vi "SR6-NC Inverse Kinematics.vi"(8 "error in (no error)":errorcluster, 10 "end effector transform":T1, 11 "SR6-NC Arm in":refnum<class "SR6-NC Arm.lvclass">) -> (0 "error out":errorcluster, 1 "number of valid solutions":i32, 2 "joint positions":T1, 3 "SR6-NC Arm out":refnum<class "SR6-NC Arm.lvclass">)   [LabVIEW 2013, in "SR6-NC Arm.lvclass"]
uses:
  SR6-NC Arm.lvclass
  <vilib>/Analysis/Matrix/Datatypes/RealMatrix.ctl
  <vilib>/robotics/Kinematics/Link/NI_Robotics_Link.lvclass/NI_Robotics_Link.ctl
  <vilib>/Analysis/baseanly.llb/Real A x B.vi
  <vilib>/Analysis/baseanly.llb/A x Vector.vi
  <vilib>/Analysis/coordinate.llb/Wrap Angle (scalar).vi
  <vilib>/Analysis/_algsub.llb/Real Vector Norm.vi
  <vilib>/Analysis/7linalg.llb/Real Transpose Matrix.vi
  <vilib>/Analysis/baseanly.llb/Real Inverse Matrix.vi
  <vilib>/robotics/Kinematics/Robot/NI_Robotics_Serial Robot Arm.lvclass
  <vilib>/robotics/Kinematics/Link/NI_Robotics_Link.lvclass
  <vilib>/Analysis/NI_AALBase.lvlib
  <vilib>/robotics/Kinematics/NI_Kinematics.lvlib
  <vilib>/Analysis/NI_AALPro.lvlib
  <vilib>/Analysis/NI_AAL_Angle.lvlib
  <vilib>/Analysis/coordinate.llb/Euler Rotation Order.ctl
  <vilib>/Analysis/Matrix/NI_Matrix.lvlib
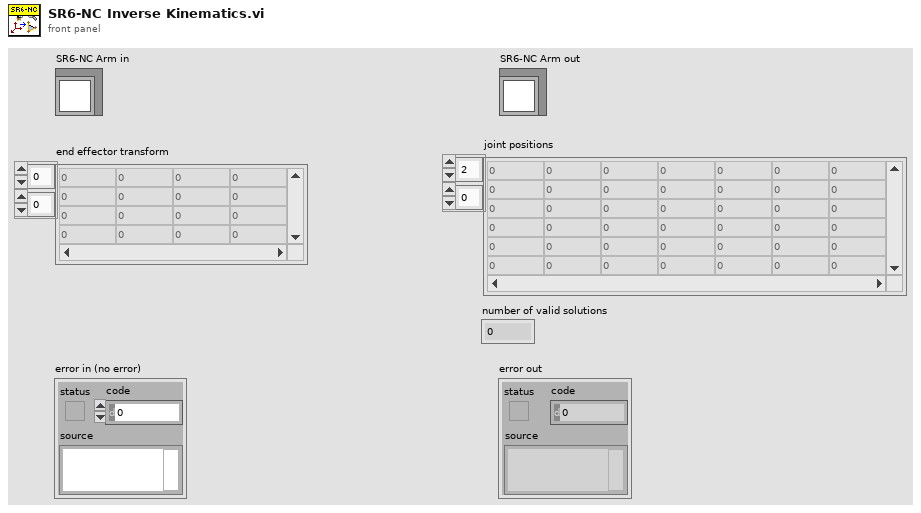
[diagram p1: front panel]
types:
  T1 = typedef "NI_Matrix.lvlib/RealMatrix.ctl" = dbl[][]
  T2 = typedef "NI_AALPro.lvlib/Euler Rotation Order.ctl" = u16
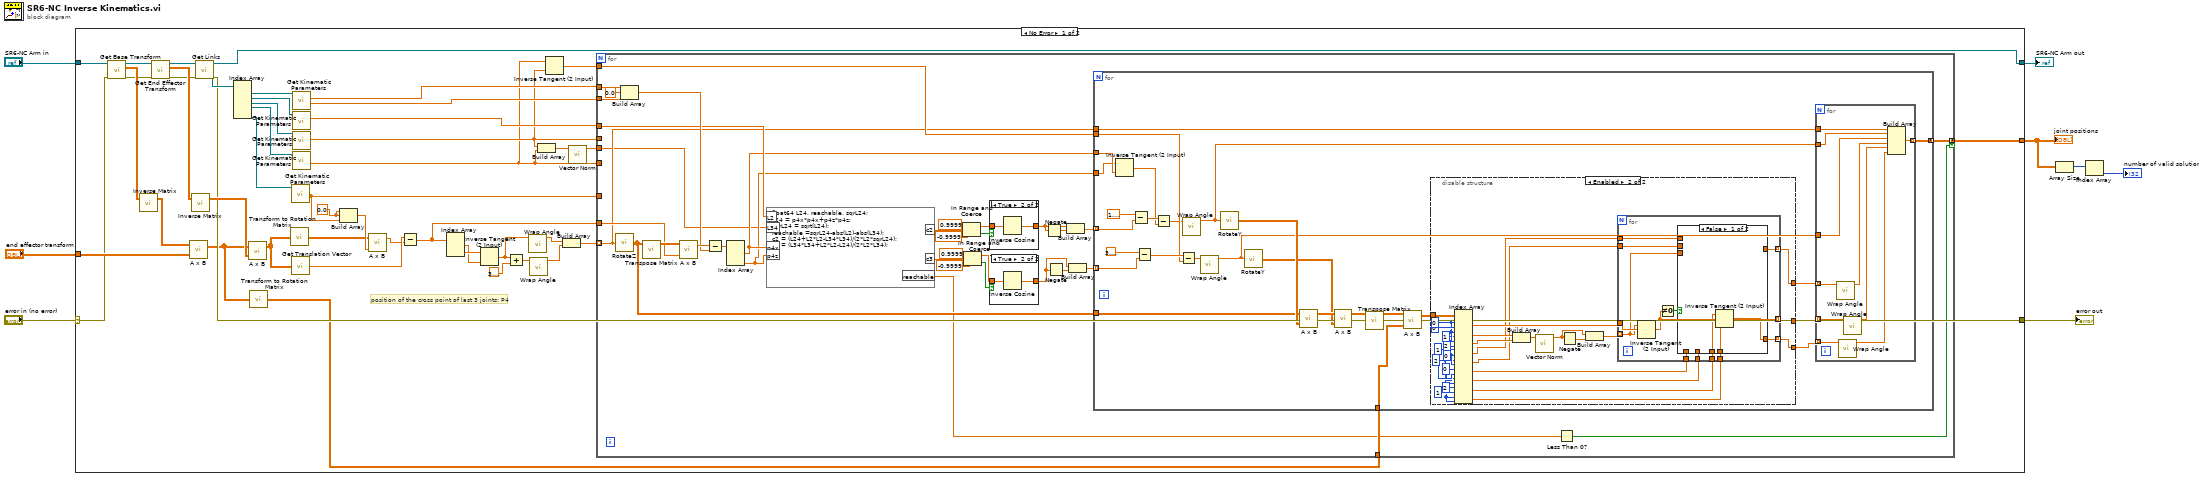
[diagram p0: block diagram]
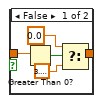
[diagram p2: hidden frame]
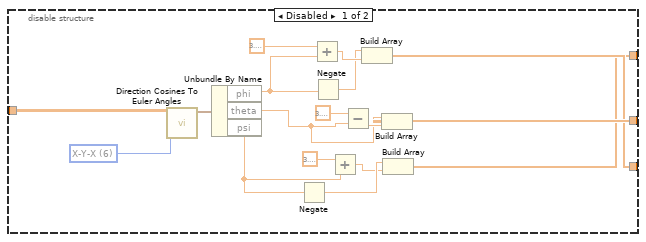
[diagram p3: hidden frame]
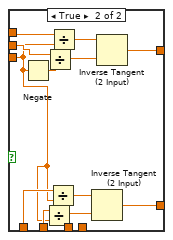
[diagram p4: hidden frame]
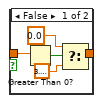
[diagram p5: hidden frame]
diagram:
  n1 = case shown="No Error" "error in (no error)" {
    selector: "error in (no error)" -> [w21 w213]
    tunnel: [w20 w213] -> w7
    tunnel: [w22 w212] -> w5
    tunnel: "SR6-NC Arm in" -> [w52 w212]
    tunnel: "end effector transform" -> [w43 _]
    tunnel: [w23 _] -> w3
    frame No Error {
      w10 = 0.0 ("element")
      # "position of the cross point of last 3 joints: P4"
      n2 = call <vilib>:"Get Base Transform.vi"("error in (no error)"=w21, "serial arm in"=w52) -> ("error out"=w45:errorcluster, "base transform"=w47:T1, "serial arm out"=w51:refnum<class "SR6-NC Arm.lvclass">)  [unwired: 7 in]
      n3 = call-poly <vilib>:"Inverse Matrix.vi"("Input Matrix"=w47) -> ("Inverse Matrix"=w49:T1)  [unwired: 1 in, 1 out]
      n4 = call <vilib>:"Get End Effector Transform.vi"("error in (no error)"=w45, "serial arm in"=w51) -> ("error out"=w44:errorcluster, "end effector transform"=w46:T1, "serial arm out"=w50:refnum<class "SR6-NC Arm.lvclass">)  [unwired: 7 in]
      n5 = call-poly <vilib>:"A x B.vi"("B"=w43, "A"=w49) -> ("A x B"=w12:T1)  [unwired: 1 out]
      n6 = call-poly <vilib>:"Inverse Matrix.vi"("Input Matrix"=w46) -> ("Inverse Matrix"=w48:T1)  [unwired: 1 in, 1 out]
      n7 = call <vilib>:"Get Links.vi"("error in (no error)"=w44, "serial arm in"=w50) -> ("error out"=w20:errorcluster, "links"=w54:refnum<class "NI_Robotics_Link.lvclass">[], "serial arm out"=w22:refnum<class "SR6-NC Arm.lvclass">)  [unwired: 7 in]
      n8 = Index Array(array=w54) -> (element #1=w53:refnum<class "NI_Robotics_Link.lvclass">, element #2=w35:refnum<class "NI_Robotics_Link.lvclass">, element #3=w34:refnum<class "NI_Robotics_Link.lvclass">, element #4=w33:refnum<class "NI_Robotics_Link.lvclass">, element #6=w32:refnum<class "NI_Robotics_Link.lvclass">)  [unwired: 6 in, 1 out]
      n9 = call-poly <vilib>:"A x B.vi"("B"=w48, "A"=w12) -> ("A x B"=w42:T1)  [unwired: 1 out]
      n10 = call <vilib>:"Transform to Rotation Matrix.vi"("transform"=w12) -> ("rotation matrix"=w11:T1)
      n11 = call <vilib>:"Transform to Rotation Matrix.vi"("transform"=w42) -> ("rotation matrix"=w13:T1)
      n12 = call <vilib>:"Get Translation Vector.vi"("transform"=w42) -> ("translation vector"=w30:dbl[])
      n13 = call <vilib>:"Get Kinematic Parameters.vi"("NI_Robotics_Link in"=w32) -> ("Offset Distance"=w9:dbl)  [unwired: 6 in, 4 out]
      n14 = call <vilib>:"Get Kinematic Parameters.vi"("NI_Robotics_Link in"=w35) -> ("Length"=w27:dbl)  [unwired: 6 in, 4 out]
      n15 = call <vilib>:"Get Kinematic Parameters.vi"("NI_Robotics_Link in"=w33) -> ("Offset Distance"=w16:dbl)  [unwired: 6 in, 4 out]
      n16 = call <vilib>:"Get Kinematic Parameters.vi"("NI_Robotics_Link in"=w53) -> ("Offset Distance"=w18:dbl, "Length"=w19:dbl)  [unwired: 6 in, 3 out]
      n17 = call <vilib>:"Get Kinematic Parameters.vi"("NI_Robotics_Link in"=w34) -> ("Length"=w17:dbl)  [unwired: 6 in, 4 out]
      n18 = Build Array(w10, w10, w9) -> (w31:dbl[])
      n19 = call-poly <vilib>:"A x B.vi"("Vector"=w31, "A"=w13) -> ("A x Vector"=w29:dbl[])  [unwired: 1 out]
      n20 = Subtract(x=w30, y=w29) -> (x-y=w28:dbl[])
      n21 = Index Array(array=w28) -> (element #1=w40:dbl, element #2=w41:dbl)  [unwired: 3 in, 1 out]
      n22 = Inverse Tangent (2 Input)(1:w40, 2:w41) -> (0:w24:dbl)
      n23 = Add(x=w24, y=3.141592653589793) -> (x+y=w38:dbl)
      n24 = call-poly <vilib>:"Wrap Angle.vi"("angle in"=w24) -> ("angle out"=w25:dbl)  [unwired: 9 in, 1 out]
      n25 = call-poly <vilib>:"Wrap Angle.vi"("angle in"=w38) -> ("angle out"=w37:dbl)  [unwired: 9 in, 1 out]
      n26 = Build Array(w17, w16) -> (w15:dbl[])
      n27 = Inverse Tangent (2 Input)(1:w17, 2:w16) -> (0:w26:dbl)
      n28 = Build Array(w25, w37) -> (w36:dbl[])
      n29 = call-poly <vilib>:"Vector Norm.vi"("Input Vector"=w15) -> ("norm"=w14:dbl)  [unwired: 9 in, 1 out]
      n30 = for {
        tunnel: w36 -> [w59] mode=indexing
        tunnel: w18 -> [w85]
        tunnel: w19 -> [w86]
        tunnel: w27 -> [w81]
        tunnel: w17 -> [_]
        tunnel: w16 -> [_]
        tunnel: w9 -> [_]
        tunnel: w28 -> [w88]
        tunnel: w26 -> [w62]
        tunnel: w11 -> [w60]
        tunnel: [w58] -> w23 mode=concatenating if=w56
        tunnel: w14 -> [w55]
        n31 = call <vilib>:"RotateZ.vi"("theta"=w59) -> ("rotation matrix"=w61:T1)
        n32 = Build Array(w86, 0.0 ("element"), w85) -> (w83:dbl[])
        n33 = call-poly <vilib>:"Transpose Matrix.vi"("Input Matrix"=w61) -> ("Matrix Transpose"=w89:T1)  [unwired: 9 in, 1 out]
        n34 = call-poly <vilib>:"A x B.vi"("Vector"=w88, "A"=w89) -> ("A x Vector"=w87:dbl[])  [unwired: 1 out]
        n35 = Subtract(x=w87, y=w83) -> (x-y=w82:dbl[])
        n36 = Index Array(array=w82) -> (element #1=w72:dbl, element #3=w71:dbl)  [unwired: 3 in, 1 out]
        n37 = formula code="float64 L24, reachable, sqrL24;\nL24 = p4x*p4x+p4z*p4z;\nsqrL24 = sqrt(L24);\nreachable =sqrL24-abs(L2)-abs(L34);\nc2 = (L24+L2*L2-L34*L34)/(2*L2*sqrL24);\nc3 = (L34*L34+L2*L2-L24)/(2*L2*L34);"("p4x"=w72, "p4z"=w71, "L2"=w81, "L34"=w55) -> ("c2"=w76:dbl, "reachable"=w57:dbl, "c3"=w66:dbl)
        n38 = In Range and Coerce(upper limit=0.9999, x=w76, lower limit=-0.9999) -> (coerced(x)=w77:dbl, In Range?=w78:bool)
        n39 = In Range and Coerce(upper limit=0.9999, x=w66, lower limit=-0.9999) -> (coerced(x)=w67:dbl, In Range?=w68:bool)
        n40 = case shown="True" w78 {
          tunnel: w77 -> [w209 w211]
          tunnel: [w205 w210] -> w74
          frame False {
            n41 = Greater Than 0?(x=w209) -> (x > 0?=w208:bool)
            n42 = Select(t=0.0, s=w208, f=3.141592653589793) -> (s? t:f=w205:dbl)
          }
          frame True {
            n43 = Inverse Cosine(1:w211) -> (0:w210:dbl)
          }
        }
        n44 = case shown="True" w68 {
          tunnel: w67 -> [w94 w96]
          tunnel: [w90 w95] -> w64
          frame False {
            n45 = Greater Than 0?(x=w94) -> (x > 0?=w93:bool)
            n46 = Select(t=0.0, s=w93, f=3.141592653589793) -> (s? t:f=w90:dbl)
          }
          frame True {
            n47 = Inverse Cosine(1:w96) -> (0:w95:dbl)
          }
        }
        n48 = Negate(x=w74) -> (-x=w75:dbl)
        n49 = Negate(x=w64) -> (-x=w65:dbl)
        n50 = Build Array(w74, w75) -> (w73:dbl[])
        n51 = Build Array(w64, w65) -> (w63:dbl[])
        n52 = for {
          tunnel: w73 -> [w122] mode=indexing
          tunnel: w72 -> [w121]
          tunnel: w71 -> [w120]
          tunnel: w63 -> [w116] mode=indexing
          tunnel: w62 -> [w114]
          tunnel: w61 -> [w97]
          tunnel: w60 -> [w108]
          tunnel: w59 -> [w101]
          tunnel: [w98] -> w58 mode=concatenating
          n53 = Inverse Tangent (2 Input)(1:w121, 2:w120) -> (0:w118:dbl)
          n54 = Subtract(x=1.5707963267948966, y=w122) -> (x-y=w119:dbl)
          n55 = Subtract(x=3.141592653589793, y=w116) -> (x-y=w115:dbl)
          n56 = Subtract(x=w119, y=w118) -> (x-y=w106:dbl)
          n57 = Subtract(x=w115, y=w114) -> (x-y=w105:dbl)
          n58 = call-poly <vilib>:"Wrap Angle.vi"("angle in"=w106) -> ("angle out"=w100:dbl)  [unwired: 9 in, 1 out]
          n59 = call-poly <vilib>:"Wrap Angle.vi"("angle in"=w105) -> ("angle out"=w99:dbl)  [unwired: 9 in, 1 out]
          n60 = call <vilib>:"RotateY.vi"("theta"=w100) -> ("rotation matrix"=w113:T1)
          n61 = call <vilib>:"RotateY.vi"("theta"=w99) -> ("rotation matrix"=w111:T1)
          n62 = call-poly <vilib>:"A x B.vi"("B"=w113, "A"=w97) -> ("A x B"=w112:T1)  [unwired: 1 out]
          n63 = call-poly <vilib>:"A x B.vi"("B"=w111, "A"=w112) -> ("A x B"=w110:T1)  [unwired: 1 out]
          n64 = call-poly <vilib>:"Transpose Matrix.vi"("Input Matrix"=w110) -> ("Matrix Transpose"=w109:T1)  [unwired: 9 in, 1 out]
          n65 = call-poly <vilib>:"A x B.vi"("B"=w108, "A"=w109) -> ("A x B"=w107:T1)  [unwired: 1 out]
          n66 = disable-structure shown="Enabled" {
            disable-tunnel: w107 -> [w140 w167]
            disable-tunnel: [w124 w151] -> w104
            disable-tunnel: [w132 w155] -> w103
            disable-tunnel: [w125 w145] -> w102
            frame Disabled {
              w139 = T2 6 items=["X-Y-Z", "X-Z-Y", "Y-X-Z", "Y-Z-X", "Z-X-Y", "Z-Y-X", "X-Y-X", "X-Z-X", "Y-X-Y", "Y-Z-Y", "Z-X-Z", "Z-Y-Z"] ("rotation order")
              n67 = call <vilib>:"Direction Cosines To Euler Angles.vi"("rotation order"=w139, "Direction Cosines"=w140) -> ("Euler Angles"=w138:cluster{"phi":dbl, "theta":dbl, "psi":dbl})  [unwired: 8 in, 1 out]
              n68 = Unbundle By Name(w138) -> ("phi"=w136:dbl, "theta"=w126:dbl, "psi"=w133:dbl)
              n69 = Negate(x=w133) -> (-x=w128:dbl)
              n70 = Add(x=3.141592653589793, y=w136) -> (x+y=w131:dbl)
              n71 = Negate(x=w136) -> (-x=w130:dbl)
              n72 = Add(x=3.141592653589793, y=w133) -> (x+y=w127:dbl)
              n73 = Subtract(x=3.141592653589793, y=w126) -> (x-y=w129:dbl)
              n74 = Build Array(w130, w131) -> (w125:dbl[])
              n75 = Build Array(w126, w129) -> (w132:dbl[])
              n76 = Build Array(w128, w127) -> (w124:dbl[])
            }
            frame Enabled {
              w143 = 2 ("index (row)")
              w149 = 0 ("index (row)")
              w148 = 2 ("index (row)")
              w154 = 0 ("disabled index (col)")
              w150 = 1 ("index (row)")
              w165 = 0 ("index (row)")
              n77 = Index Array(array=w167, index (row) #1=w165, index (col) #1=0 ("disabled index (col)"), index (row) #2=w165, index (col) #2=1 ("disabled index (col)"), index (row) #3=w165, index (col) #3=2 ("disabled index (col)"), index (row) #4=w150, index (col) #4=w154, index (row) #5=w148, index (col) #5=w154, index (row) #6=w149, index (col) #6=w150, index (row) #7=w149, index (col) #7=w148, index (row) #8=w143, index (col) #8=1 ("disabled index (col)"), index (row) #9=w143, index (col) #9=w143) -> (element #1=w156:dbl, element #2=w161:dbl, element #3=w162:dbl, element #4=w153:dbl, element #5=w152:dbl, element #6=w147:dbl, element #7=w146:dbl, element #8=w142:dbl, element #9=w141:dbl)
              n78 = Build Array(w161, w162) -> (w160:dbl[])
              n79 = call-poly <vilib>:"Vector Norm.vi"("Input Vector"=w160) -> ("norm"=w158:dbl)  [unwired: 9 in, 1 out]
              n80 = Negate(x=w158) -> (-x=w159:dbl)
              n81 = Build Array(w158, w159) -> (w157:dbl[])
              n82 = for {
                tunnel: w157 -> [w174] mode=indexing
                tunnel: w156 -> [w179]
                tunnel: [w178] -> w155 mode=indexing
                tunnel: w153 -> [w176]
                tunnel: w152 -> [w175]
                tunnel: [w173] -> w151 mode=indexing
                tunnel: w147 -> [w172]
                tunnel: w146 -> [w171]
                tunnel: [w170] -> w145 mode=indexing
                tunnel: w142 -> [w169]
                tunnel: w141 -> [w168]
                n83 = Inverse Tangent (2 Input)(1:w179, 2:w174) -> (0:w178:dbl)
                n84 = Not Equal To 0?(x=w178) -> (x != 0?=w177:bool)
                n85 = case shown="False" w177 {
                  tunnel: w176 -> [_ w194]
                  tunnel: w175 -> [_ w193]
                  tunnel: w174 -> [_ w186]
                  tunnel: [_ w189] -> w173
                  tunnel: w172 -> [_ w188]
                  tunnel: w171 -> [_ w187]
                  tunnel: [w180 w183] -> w170
                  tunnel: w169 -> [w182 _]
                  tunnel: w168 -> [w181 _]
                  frame False {
                    n86 = Inverse Tangent (2 Input)(1:w181, 2:w182) -> (0:w180:dbl)
                  }
                  frame True {
                    n87 = Negate(x=w186) -> (-x=w192:dbl)
                    n88 = Divide(x=w187, y=w186) -> (x/y=w184:dbl)
                    n89 = Divide(x=w193, y=w192) -> (x/y=w190:dbl)
                    n90 = Divide(x=w188, y=w186) -> (x/y=w185:dbl)
                    n91 = Divide(x=w194, y=w186) -> (x/y=w191:dbl)
                    n92 = Inverse Tangent (2 Input)(1:w184, 2:w185) -> (0:w183:dbl)
                    n93 = Inverse Tangent (2 Input)(1:w190, 2:w191) -> (0:w189:dbl)
                  }
                }
              }
            }
          }
          n94 = for {
            tunnel: w104 -> [w204] mode=indexing
            tunnel: w103 -> [w195] mode=indexing
            tunnel: w102 -> [w203] mode=indexing
            tunnel: w101 -> [w202]
            tunnel: w100 -> [w201]
            tunnel: w99 -> [w200]
            tunnel: [w196] -> w98 mode=indexing
            n95 = call-poly <vilib>:"Wrap Angle.vi"("angle in"=w204) -> ("angle out"=w199:dbl)  [unwired: 9 in, 1 out]
            n96 = call-poly <vilib>:"Wrap Angle.vi"("angle in"=w203) -> ("angle out"=w197:dbl)  [unwired: 9 in, 1 out]
            n97 = call-poly <vilib>:"Wrap Angle.vi"("angle in"=w195) -> ("angle out"=w198:dbl)  [unwired: 9 in, 1 out]
            n98 = Build Array(w202, w201, w200, w199, w198, w197) -> (w196:dbl[])
          }
        }
        n99 = Less Than 0?(x=w57) -> (x < 0?=w56:bool)
      }
    }
    frame Error {
    }
  }
  "error out" <- w7
  "SR6-NC Arm out" <- w5
  "joint positions" <- w3
  n100 = Array Size(array=w3) -> (size(s)=w2:i32[])
  n101 = Index Array(array=w2) -> (element=→"number of valid solutions":i32)  [unwired: 1 in]
